vi "Get_Aspect_Ratio.vi"(9 "# Buses":i32) -> (1 "Aspect ratio":dbl)   [LabVIEW 2010]
doc: "This VI gets the aspect ratio for the circuit considering the number of buses defined on the buscoords file.\n\nCreated by Davis Montenegro\n17-05-2017"
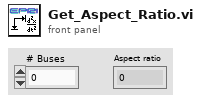
[diagram p1: front panel]
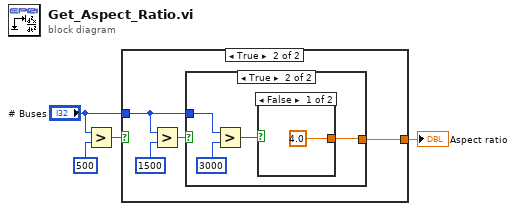
[diagram p0: block diagram]
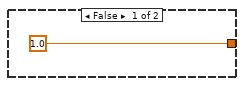
[diagram p2: hidden frame]
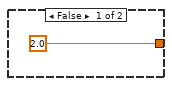
[diagram p3: hidden frame]
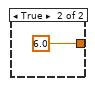
[diagram p4: hidden frame]
diagram:
  n1 = Greater?(x="# Buses", y=500) -> (0:w3:bool)
  n2 = case shown="True" w3 {
    tunnel: [1.0 w7] -> w1
    tunnel: "# Buses" -> [_ w6]
    frame False {
    }
    frame True {
      n3 = Greater?(x=w6, y=1500) -> (0:w8:bool)
      n4 = case shown="True" w8 {
        tunnel: [2.0 w11] -> w7
        tunnel: w6 -> [_ w14]
        frame False {
        }
        frame True {
          n5 = Greater?(x=w14, y=3000) -> (0:w12:bool)
          n6 = case shown="False" w12 {
            tunnel: [4.0 6.0] -> w11
            frame False {
            }
            frame True {
            }
          }
        }
      }
    }
  }
  "Aspect ratio" <- w1
